vi "ConfigECUInfo.vi"(8 "error in (no error)":errorcluster, 10 "Parttype":refnum<vi>, 11 "ECU Info":T1) -> (0 "error out":errorcluster, 2 "ECU Info":T1, 3 "change?":bool)   [LabVIEW 2014]
uses:
  typedefs/parttype.ctl
  <vilib>/Utility/config.llb/Write Key (String).vi
  <vilib>/Utility/config.llb/NI_LVConfig.lvlib
panel:
  in  "Cancel":bool
  in  "OK":bool
  # "Config ECU Info"
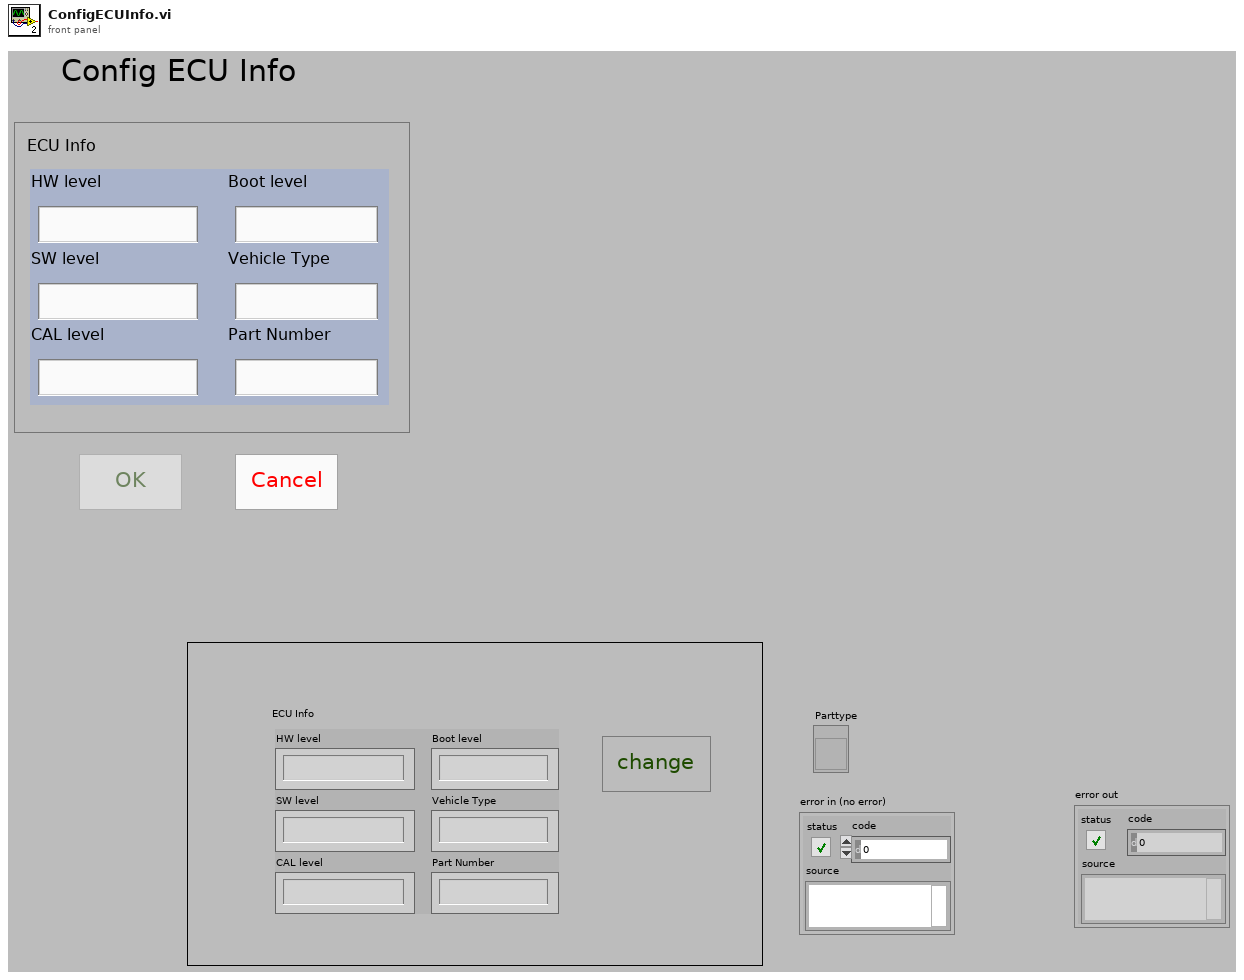
[diagram p1: front panel]
types:
  T1 = cluster{"HW level":string, "SW level":string, "CAL level":string, "Boot level":string, "Vehicle Type":string, "Part Number":string}
  T2 = enum8{"Enabled", "Disabled", "Disabled and Grayed Out"}
  T3 = typedef "parttype.ctl" = enum16{"NMS", "B-SUV"}
  T4 = typedef "NI_LVConfig.lvlib/Config Data RefNum.ctl" = refnum<k1>
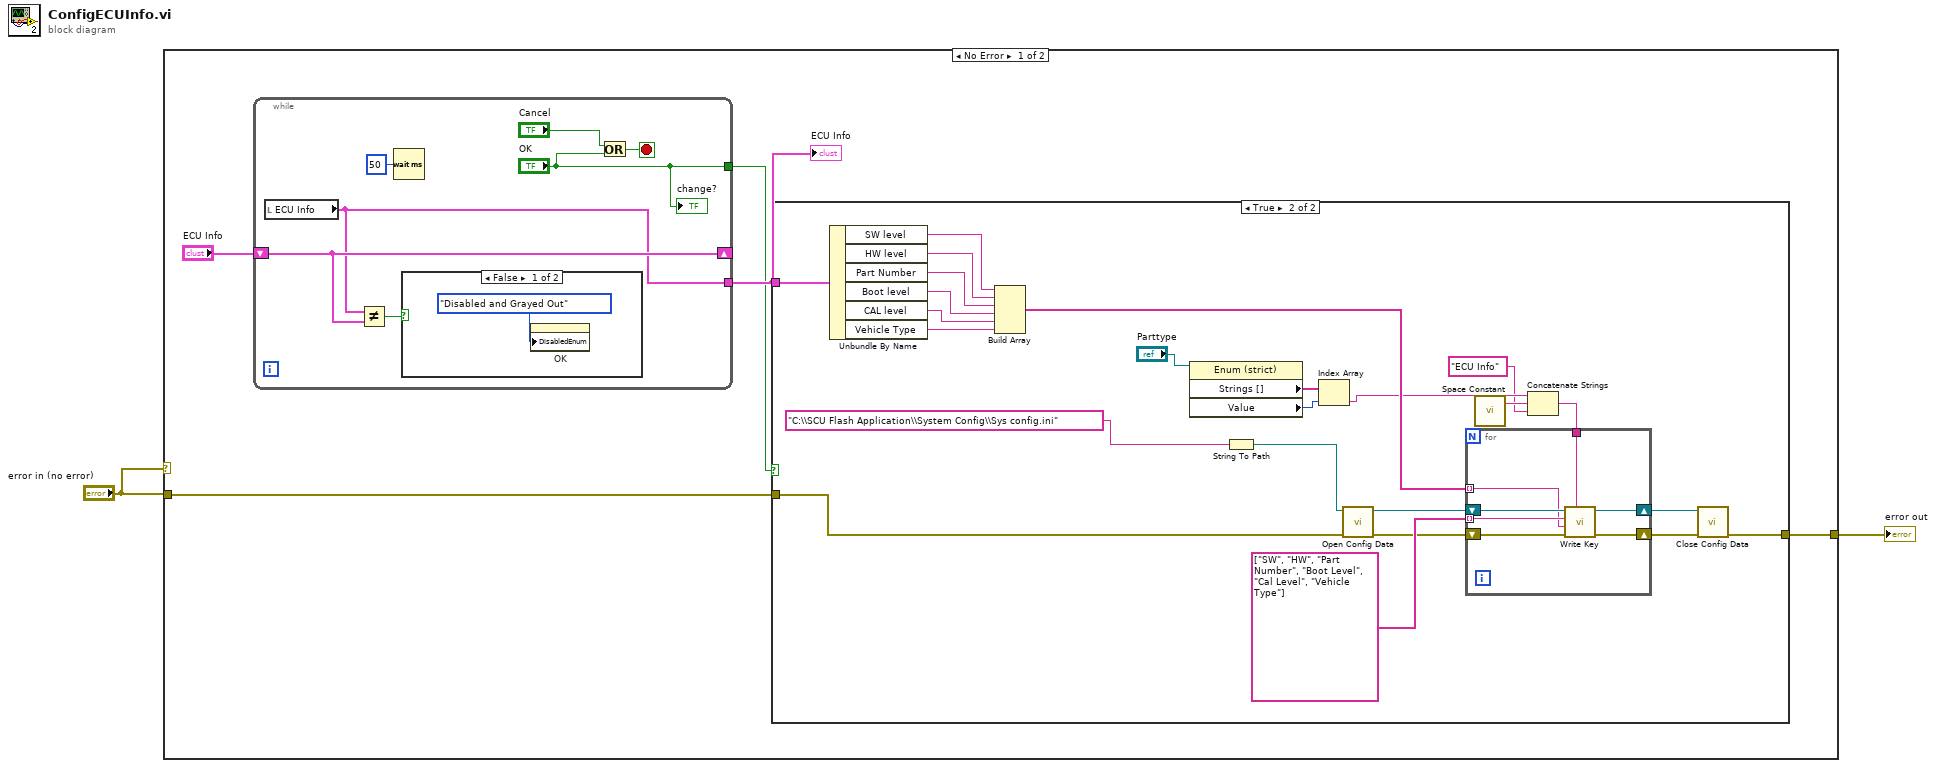
[diagram p0: block diagram]
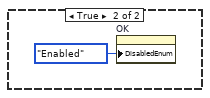
[diagram p3: hidden frame]
diagram:
  n1 = case shown="No Error" "error in (no error)" {
    tunnel: [w4 w49] -> w2
    tunnel: "error in (no error)" -> [w3 w49]
    frame No Error {
      n2 = while {
        shift-right: [w42] -> _
        shift-left: "ECU Info" -> [w42]
        tunnel: [w41] -> w6
        tunnel: ["OK"] -> w5
        stop <- w44 stop-if-true
        n3 = local read "ECU Info"() -> (w41:T1)
        n4 = Not Equal?(x=w41, y=w42) -> (x != y?=w43:bool)
        n5 = Wait (ms)(milliseconds to wait=u32 50) -> ()  [unwired: 1 out]
        n6 = case shown="False" w43 {
          frame False {
            n7 = property on="OK" class="Bool"("DisabledEnum"=T2."Disabled and Grayed Out" ("Disabled")) -> ()  [unwired: 2 in, 2 out]
          }
          frame True {
            n8 = property on="OK" class="Bool"("DisabledEnum"=T2."Enabled" ("Disabled")) -> ()  [unwired: 2 in, 2 out]
          }
        }
        n9 = Or(x="Cancel", y="OK") -> (x .or. y?=w44:bool)
        "change?" <- "OK"
      }
      "ECU Info" <- w6
      n10 = case shown="True" w5 {
        tunnel: w6 -> [_ w26]
        tunnel: [w8 w18] -> w4
        tunnel: w3 -> [w8 w17]
        frame False {
        }
        frame True {
          n11 = Unbundle By Name(w26) -> ("SW level"=w25:string, "HW level"=w24:string, "Part Number"=w23:string, "Boot level"=w22:string, "CAL level"=w21:string, "Vehicle Type"=w20:string)
          n12 = Build Array(w25, w24, w23, w22, w21, w20) -> (w19:string[])
          n13 = property class="Enum (strict)"(reference="Parttype") -> ("Strings []"=w14:string[], "Value"=w15:T3)  [unwired: 1 in, 2 out]
          n14 = String To Path(string="C:\\SCU Flash Application\\System Config\\Sys config.ini" ("name or relative path")) -> (path=w32:path)
          n15 = Index Array(array=w14, index=w15) -> (element=w12:string)
          n16 = call <vilib>:"Open Config Data.vi"("error in (no error)"=w17, "configuration file path"=w32) -> ("error out"=w29:errorcluster, "refnum"=w28:T4)  [unwired: 7 in, 1 out]
          n17 = call <vilib>:"Space Constant.vi"() -> ("String"=w11:string)
          n18 = Concatenate Strings(w12, w11, "ECU Info" ("section")) -> (w9:string)
          n19 = for {
            tunnel: string[] ["SW", "HW", "Part Number", "Boot Level", "Cal Level", "Vehicle Type"] -> [w37] mode=indexing
            shift-right: [w36] -> w30
            shift-left: w28 -> [w39]
            shift-right: [w35] -> w27
            shift-left: w29 -> [w38]
            tunnel: w19 -> [w34] mode=indexing
            tunnel: w9 -> [w33]
            n20 = call-poly <vilib>:"Write Key.vi"("section"=w33, "error in (no error)"=w38, "value"=w34, "key"=w37, "refnum"=w39) -> ("error out"=w35:errorcluster, "refnum out"=w36:T4)  [unwired: 4 in, 1 out]
          }
          n21 = call <vilib>:"Close Config Data.vi"("error in (no error)"=w27, "refnum"=w30) -> ("error out"=w18:errorcluster)  [unwired: 8 in, 1 out]
        }
      }
    }
    frame Error {
    }
  }
  "error out" <- w2
